vi "Prueba.vi"() -> ()   [LabVIEW 2017]
uses:
  <vilib>/picture/3D Picture Control/NI_3D Picture Control.lvlib
panel:
  in  "Mundo":path
  out "3D Picture":refnum<vi>(3d-picture)
  in  "Stop Button":bool
  in  "Objetos":path
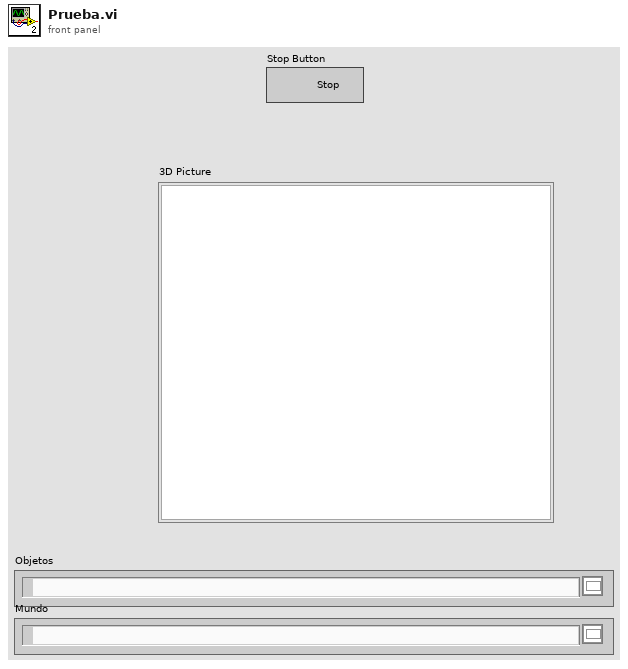
[diagram p1: front panel]
types:
  T1 = enum16{"open", "replace", "create", "open or create", "replace or create", "replace or create with confirmation"}
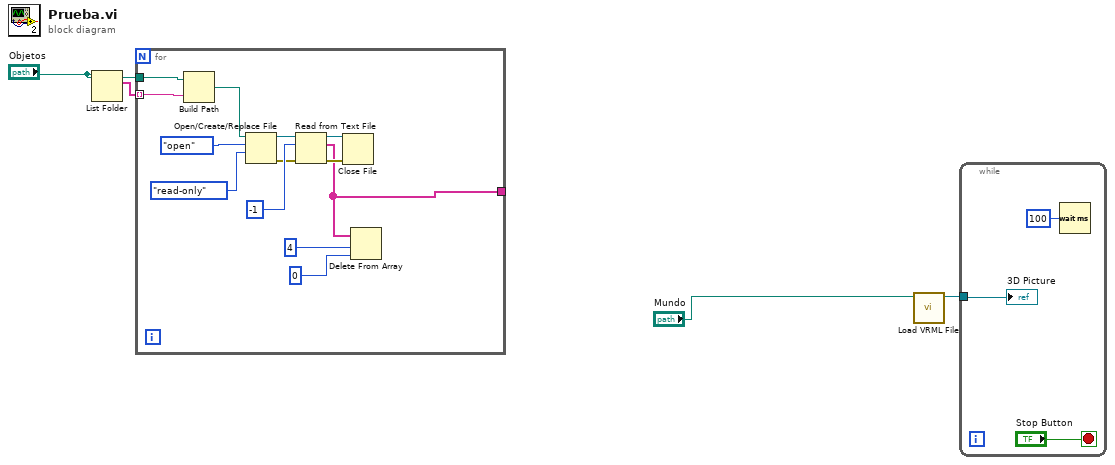
[diagram p0: block diagram]
diagram:
  n1 = List Folder(path="Objetos") -> (filenames=w4:string[])  [unwired: 3 in, 3 out]
  n2 = for {
    tunnel: w4 -> [w17] mode=indexing
    tunnel: "Objetos" -> [w16]
    tunnel: [w5] -> _
    n3 = Build Path(base path=w16, name or relative path=w17) -> (appended path=w15:path)
    n4 = Open/Create/Replace File(file path (use dialog)=w15, operation (0:open)=T1."open", access (0:read/write)=enum16{"read/write", "read-only", "write-only"}."read-only") -> (refnum out=w12:refnum<file>, error out=w10:errorcluster)  [unwired: 3 in, 1 out]
    n5 = Read from Text File(file (use dialog)=w12, count=-1, error in=w10) -> (refnum out=w8:refnum<file>, text=w5:string[], error out=w9:errorcluster)  [unwired: 1 in, 1 out]
    n6 = Close File(refnum=w8, error in=w9) -> ()  [unwired: 2 out]
    n7 = Delete From Array(array=w5, length=4, index=0) -> ()  [unwired: 2 out]
  }
  n8 = call <vilib>:"Load VRML File.vi"("Path"="Mundo") -> ("Scene:Read Scene File"=w2:refnum<vi>)  [unwired: 9 in, 1 out]
  n9 = while {
    tunnel: w2 -> [w18]
    stop <- "Stop Button" stop-if-true
    n10 = Wait (ms)(milliseconds to wait=u32 100) -> ()  [unwired: 1 out]
    "3D Picture" <- w18
  }
